vi "State_Machine.vi"(8 "error in (no error)":errorcluster caption="entrée d'erreur (pas d'erreur)", 11 "Get_Voltage en entrée":refnum<class "Start_Blink_Relay.lvclass">) -> (0 "error out":errorcluster caption="sortie d'erreur", 2 "Json_String":string, 3 "Get_Voltage en sortie":refnum<class "Start_Blink_Relay.lvclass">)   [LabVIEW 2020, in "Library Test.lvlib" / "Start_Blink_Relay.lvclass"]
uses:
  Start_Blink_Relay.lvclass
  C:/Users/ngarcin/OneDrive - Altyor/Standard TB/Suite TB45/Class/Test/Test (Default)/Test (Default).lvclass
  Commun VI/TypeDef/Variable Printable.ctl
  <vilib>/Platform/TimedLoop/XDataNode/timing_clust.ctl
  <vilib>/Platform/TimedLoop/XDataNode/nitl_modes.ctl
  <vilib>/Platform/TimedLoop/XDataNode/wakeup.ctl
  Commun VI/TypeDef/Commande Relay_Board/Data_Write_Relay_Board.ctl
  Start_Blink_Relay.lvclass/Start_Blink_Relay.ctl
  JSON API/Variant JSON/Variant to JSON.vi
  JSON API/JSON Value/Get Item by name array.vi
  Instrument/Instrument (Default)/Class Instrument (Default).lvclass
  <vilib>/Platform/TimedLoop/XDataNode/XDataNode.xnode
  JSON API/JSON Value/JSON Value.lvclass
  JSON API/Get Polymorphic/JSON GetSet.lvlib
  Commun VI/Library Commun.lvlib
  JSON API/Variant JSON/Variant JSON.lvlib
  <vilib>/Platform/TimedLoop/XDataNode/XDNodeRunTimeDep.lvlib
panel:
  in  "stop":bool
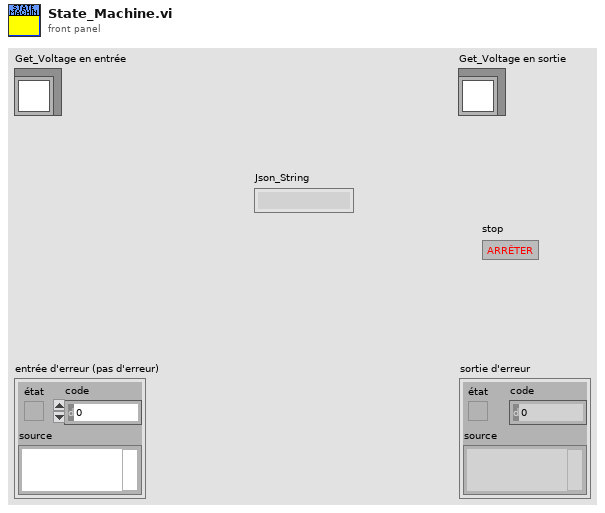
[diagram p1: front panel]
types:
  T1 = typedef "Variable Printable.ctl" = string
  T2 = enum16{"Get Variable", "Get All Variables", "Set Variable", "Delete Variable", "Delete All Variable"}
  T3 = enum16{"Disable Relay", "Write Value", "Finish"}[]
  T4 = typedef "Library Commun.lvlib/Data_Write_Relay_Board.ctl" = enum16{"Enable Relays", "Disable Relays"}
  T5 = typedef "XDNodeRunTimeDep.lvlib/timing_clust.ctl" = cluster{"Expected End [f-1]":u64, "Actual End [f-1]":u64, "Finished Late? [f-1]":bool, "Expected End [i-1]":u64, "Actual End [i-1]":u64, "Finished Late? [i-1]":bool, "Expected Start [i]":u64, "Actual Start [i]":u64, "Expected Start [f]":u64, "Actual Start [f]":u64, "Source Name":string, "Structure Name":string, "Period":i64, "Deadline":i64, "Offset":i64, "Start":i64, "Priority":i32, "Timeout":i32, "Mode":T6, "Wakeup Reason":T7, "Error":errorcluster, "Source Type":string, "Secondary Source Type":string, "Global End Time":u64, "Global Start Time":u64, "Frame Duration":u64, "Iteration Duration":u64, "Assigned CPU":i32, "I/O Scan Engine Mode":u32}
  T6 = typedef "XDNodeRunTimeDep.lvlib/nitl_modes.ctl" = enum32{"No Change", "Process missed periods, maintain original phase", "Discard missed periods, maintain original phase", "Process missed periods, ignore original phase", "Discard missed periods, ignore original phase"}
  T7 = typedef "XDNodeRunTimeDep.lvlib/wakeup.ctl" = enum32{"Normal", "Aborted", "Asynchronous wakeup", "Timing source error", "Timed loop error", "Timeout"}
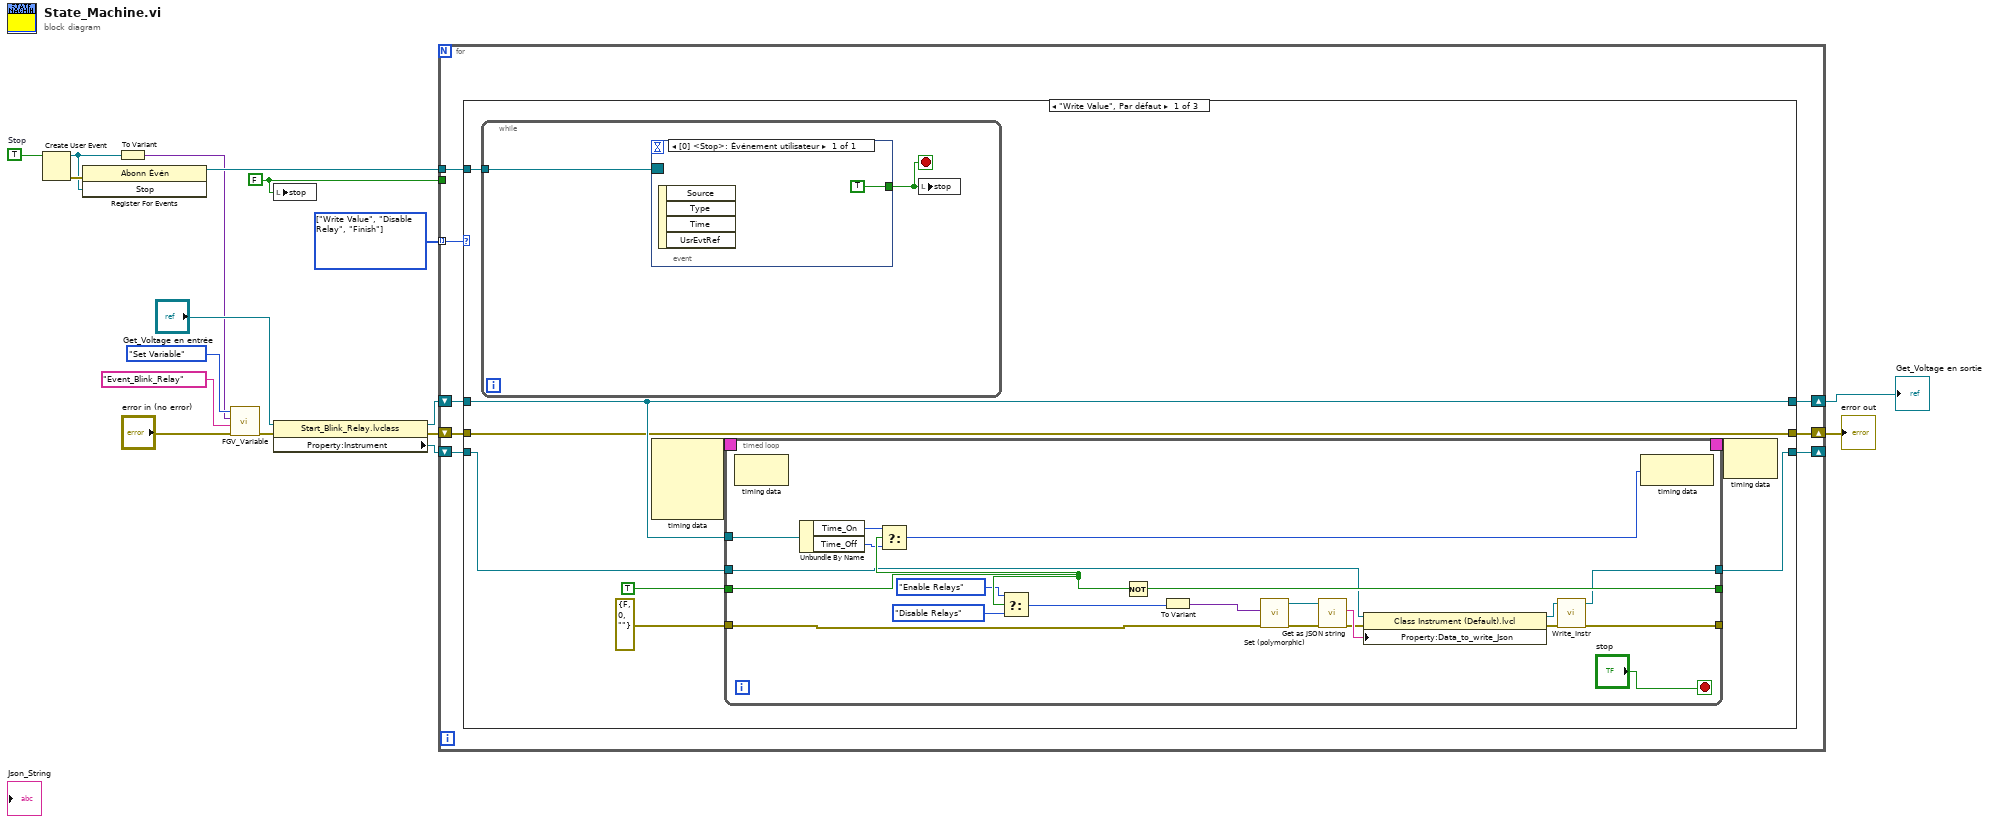
[diagram p0: block diagram]
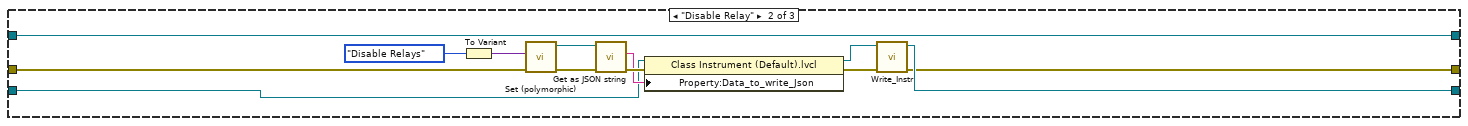
[diagram p2: hidden frame]
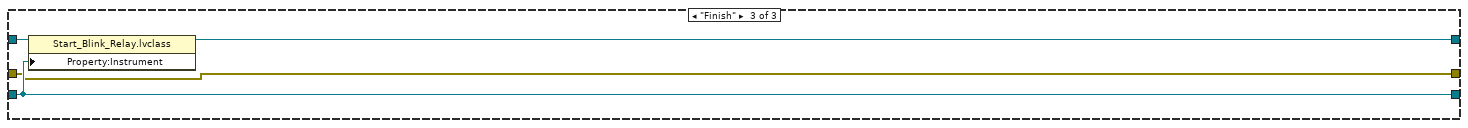
[diagram p3: hidden frame]
diagram:
  w3 = FALSE ("stop")
  w10 = TRUE  # Stop
  w16 = T3 [enum."Write Value", enum."Disable Relay", enum."Finish"] items=["Disable Relay", "Write Value", "Finish"]
  n1 = Create User Event(user event datatype=w10) -> (user event=w2:refnum<user-event>, error out=w9:errorcluster)  [unwired: 1 in]
  n2 = register-events(error in=w9, w2) -> (reference out=w6:refnum<event-registration>)  [unwired: 1 in, 1 out]
  n3 = To Variant(anything=w2) -> (Variant=w1:variant)
  n4 = call "FGV_Variable.vi"("error in (no error)"="error in (no error)", "Variable"=T1 "Event_Blink_Relay", "Data In"=w1, "Function"=T2."Set Variable") -> ("error out"=w4:errorcluster)  [unwired: 5 in, 2 out]
  n5 = local write "stop"(w3) -> ()
  n6 = property class="Start_Blink_Relay.lvclass"(reference="Get_Voltage en entrée", error in=w4) -> (reference out=w14:refnum<class "Start_Blink_Relay.lvclass">, error out=w11:errorcluster, "Property:Instrument"=w15:refnum<class "Class Instrument (Default).lvclass">)
  n7 = for {
    tunnel: w16 -> [w25] mode=indexing
    shift-right: [w23] -> _
    shift-left: w15 -> [w24]
    shift-right: [w21] -> w12
    shift-left: w14 -> [w22]
    shift-right: [w19] -> w13
    shift-left: w11 -> [w20]
    tunnel: w6 -> [w18]
    tunnel: w3 -> [_]
    n8 = case shown="\"Write Value\", Par défaut" w25 {
      tunnel: w24 -> [w33 w68 w79]
      tunnel: [w28 w66 w79] -> w23
      tunnel: w22 -> [w31 w77 w81]
      tunnel: [w31 w77 w80] -> w21
      tunnel: w20 -> [w30 w67 w78]
      tunnel: [w30 w65 w78] -> w19
      tunnel: w18 -> [w34 _ _]
      frame "Write Value", Default {
        n9 = while {
          tunnel: w34 -> [w63]
          stop <- w62 stop-if-true
          n10 = event shown="[0] <Stop>: Événement utilisateur" {
            selector: w63 -> [_]
            dyn-events: _ -> [_]
            timeout: _ -> [_]
            tunnel: [TRUE] -> w62
            event User Event {
              n11 = event-data() -> ()  [unwired: 1 in, 4 out]
            }
          }
          n12 = local write "stop"(w62) -> ()
        }
        n13 = node-c288() -> (w27:T5)  [unwired: 4 in]
        n14 = timed-loop {
          tunnel: w31 -> [w55]
          tunnel: TRUE -> [w54]
          tunnel: [w53] -> _
          tunnel: w33 -> [w52]
          tunnel: [w51] -> w28
          tunnel: errorcluster {"status"=FALSE, "code"=0, "source"=""} ("error out") -> [w50]
          tunnel: [w49] -> _
          timing: w27 -> [_]
          timing-out: [_] -> w26
          stop <- "stop" stop-if-true
          n15 = node-c288() -> ()  [unwired: 1 in, 1 out]
          n16 = Unbundle By Name(w55) -> ("Time_On"=w41:u16, "Time_Off"=w40:u16)
          n17 = Select(t=w41, s=w54, f=w40) -> (s? t:f=w35:u16)
          n18 = Select(t=Data_Write_Relay_Board."Enable Relays" ("Function"), s=w54, f=Data_Write_Relay_Board."Disable Relays" ("Function")) -> (s? t:f=w37:T4)
          n19 = Not(x=w54) -> (.not. x?=w53:bool)
          n20 = To Variant(anything=w37) -> (Variant=w47:variant)
          n21 = call-poly "Set (polymorphic).vi"("error in (no error)"=w50, "Variant"=w47) -> ("error out"=w48:errorcluster, "JSON Value out"=w46:refnum<class "JSON Value.lvclass">)  [unwired: 8 in]
          n22 = call "Get as JSON string.vi"("error in (no error)"=w48, "JSON Value in"=w46) -> ("error out"=w42:errorcluster, "<JSON>"=w45:string)  [unwired: 8 in]
          n23 = property class="Class Instrument (Default).lvcl"(reference=w52, error in=w42, "Property:Data_to_write_Json"=w45) -> (reference out=w44:refnum<class "Class Instrument (Default).lvclass">, error out=w43:errorcluster)
          n24 = call-dynamic "Write_Instr.vi"("error in (no error)"=w43, "Class Multimeter (Default) en entrée"=w44) -> ("error out"=w49:errorcluster, "Class Multimeter (Default) en sortie"=w51:refnum<class "Class Instrument (Default).lvclass">)  [unwired: 8 in]
          n25 = node-c288(w35) -> ()  [unwired: 1 out]
        }
        n26 = node-c288(w26) -> ()  [unwired: 1 out]
      }
      frame "Disable Relay" {
        n27 = To Variant(anything=Data_Write_Relay_Board."Disable Relays" ("Function")) -> (Variant=w73:variant)
        n28 = call-poly "Set (polymorphic).vi"("error in (no error)"=w67, "Variant"=w73) -> ("error out"=w72:errorcluster, "JSON Value out"=w74:refnum<class "JSON Value.lvclass">)  [unwired: 8 in]
        n29 = call "Get as JSON string.vi"("error in (no error)"=w72, "JSON Value in"=w74) -> ("error out"=w76:errorcluster, "<JSON>"=w75:string)  [unwired: 8 in]
        n30 = property class="Class Instrument (Default).lvcl"(reference=w68, error in=w76, "Property:Data_to_write_Json"=w75) -> (reference out=w71:refnum<class "Class Instrument (Default).lvclass">, error out=w69:errorcluster)
        n31 = call-dynamic "Write_Instr.vi"("error in (no error)"=w69, "Class Multimeter (Default) en entrée"=w71) -> ("error out"=w65:errorcluster, "Class Multimeter (Default) en sortie"=w66:refnum<class "Class Instrument (Default).lvclass">)  [unwired: 8 in]
      }
      frame "Finish" {
        n32 = property class="Start_Blink_Relay.lvclass"(reference=w81, "Property:Instrument"=w79) -> (reference out=w80:refnum<class "Start_Blink_Relay.lvclass">)  [unwired: 1 in, 1 out]
      }
    }
  }
  "error out" <- w13
  "Get_Voltage en sortie" <- w12
